vi "GradientVI.vi"(0 "x(m)":dbl[](array[numeric])=[-0.124, -0.174, 0.124, 0.174], 1 "erot(V/cm)":dbl=22.0, 5 "B(G)":dbl[](array[numeric])=[0.670549623135055, 0.512230952892665, 0.685842810963684, 0.53621930068775], 7 "uncertainty(G)":dbl[](array[numeric])=[0.010516573446927, 0.009705496604384, 0.010177056389311, 0.011331487675758], 9 "initial guess(A)":dbl[](array[numeric])=[0.5], 11 "error in (no error)":errorcluster, 12 "freq (Hz)":dbl=1589645.882716435) -> (4 "Fitted I(A)":dbl[](array[numeric])=[0.7805554383201968], 6 "dB(mG/cm)":dbl=66.15007442640399, 8 "Frequency(Hz)":dbl=35.75963864978995, 10 "XY Graph":cluster{"X":dbl[], "Y":dbl[]}[](graph)=[{"X"=[-0.2, -0.19798994974874373, -0.19597989949748745, -0.19396984924623117, -0.1919597989949749, -0.18994974874371862, -0.1879396984924623, -0.18592964824120603, -0.18391959798994975, -0.18190954773869347, -0.1798994974874372, -0.17788944723618091, -0.17587939698492464, -0.17386934673366836, -0.17185929648241208, -0.1698492462311558, -0.16783919597989952, -0.1658291457286432, -0.16381909547738693, -0.16180904522613065, -0.15979899497487438, -0.1577889447236181, -0.15577889447236182, -0.15376884422110554, -0.15175879396984926, -0.14974874371859298, -0.1477386934673367, -0.14572864321608042, -0.14371859296482412, -0.14170854271356784, -0.13969849246231156, -0.13768844221105528, -0.135678391959799, -0.13366834170854272, -0.13165829145728644, -0.12964824120603016, -0.12763819095477388, -0.1256281407035176, -0.12361809045226131, -0.12160804020100503, -0.11959798994974875, -0.11758793969849247, -0.11557788944723618, -0.1135678391959799, -0.11155778894472362, -0.10954773869346734, -0.10753768844221107, -0.10552763819095477, -0.1035175879396985, -0.10150753768844221, -0.09949748743718594, -0.09748743718592966, -0.09547738693467338, -0.09346733668341708, -0.0914572864321608, -0.08944723618090453, -0.08743718592964825, -0.08542713567839197, -0.08341708542713569, -0.0814070351758794, -0.07939698492462312, -0.07738693467336684, -0.07537688442211056, -0.07336683417085428, -0.07135678391959799, -0.06934673366834171, -0.06733668341708543, -0.06532663316582915, -0.06331658291457287, -0.061306532663316586, -0.05929648241206031, -0.05728643216080402, -0.05527638190954774, -0.05326633165829146, -0.05125628140703518, -0.0492462311557789, -0.04723618090452262, -0.04522613065326633, -0.043216080402010054, -0.04120603015075377, -0.03919597989949749, -0.03718592964824121, -0.035175879396984924, -0.033165829145728645, -0.031155778894472363, -0.02914572864321608, -0.0271356783919598, -0.02512562814070352, -0.023115577889447236, -0.021105527638190957, -0.019095477386934675, -0.017085427135678392, -0.015075376884422112, -0.01306532663316583, -0.011055276381909548, -0.009045226130653268, -0.007035175879396985, -0.005025125628140704, -0.0030150753768844224, -0.0010050251256281408, 0.0010050251256281408, 0.0030150753768844224, 0.005025125628140704, 0.007035175879396985, 0.009045226130653268, 0.011055276381909548, 0.01306532663316583, 0.015075376884422112, 0.017085427135678392, 0.019095477386934675, 0.021105527638190957, 0.023115577889447236, 0.02512562814070352, 0.0271356783919598, 0.02914572864321608, 0.031155778894472363, 0.033165829145728645, 0.035175879396984924, 0.03718592964824121, 0.03919597989949749, 0.04120603015075377, 0.043216080402010054, 0.04522613065326633, 0.04723618090452262, 0.0492462311557789, 0.05125628140703518, 0.05326633165829146, 0.05527638190954774, 0.05728643216080402, 0.05929648241206031, 0.061306532663316586, 0.06331658291457287, 0.06532663316582915, 0.06733668341708543, 0.06934673366834171, 0.07135678391959799, 0.07336683417085428, 0.07537688442211056, 0.07738693467336684, 0.07939698492462312, 0.0814070351758794, 0.08341708542713569, 0.08542713567839197, 0.08743718592964825, 0.08944723618090453, 0.0914572864321608, 0.09346733668341708, 0.09547738693467338, 0.09748743718592966, 0.09949748743718594, 0.10150753768844221, 0.1035175879396985, 0.10552763819095477, 0.10753768844221107, 0.10954773869346734, 0.11155778894472362, 0.1135678391959799, 0.11557788944723618, 0.11758793969849247, 0.11959798994974875, 0.12160804020100503, 0.12361809045226131, 0.1256281407035176, 0.12763819095477388, 0.12964824120603016, 0.13165829145728644, 0.13366834170854272, 0.135678391959799, 0.13768844221105528, 0.13969849246231156, 0.14170854271356784, 0.14371859296482412, 0.14572864321608042, 0.1477386934673367, 0.14974874371859298, 0.15175879396984926, 0.15376884422110554, 0.15577889447236182, 0.1577889447236181, 0.15979899497487438, 0.16180904522613065, 0.16381909547738693, 0.1658291457286432, 0.16783919597989952, 0.1698492462311558, 0.17185929648241208, 0.17386934673366836, 0.17587939698492464, 0.17788944723618091, 0.1798994974874372, 0.18190954773869347, 0.18391959798994975, 0.18592964824120603, 0.1879396984924623, 0.18994974874371862, 0.1919597989949749, 0.19396984924623117, 0.19597989949748745, 0.19798994974874373, 0.2], "Y"=[0.4343731207716029, 0.4433656420187343, 0.4523999073237652, 0.4614632556723153, 0.4705421469697098, 0.47962216308459116, 0.48868801544118295, 0.49772355973172244, 0.5067118182846725, 0.515635010574119, 0.5244745922903558, 0.5332113033105923, 0.5418252248117672, 0.5502958456549943, 0.558602138043926, 0.5667226423186786, 0.5746355605948373, 0.5823188587959173, 0.5897503764606421, 0.5969079435370565, 0.6037695032079631, 0.6103132396308245, 0.61651770932489, 0.6223619748035435, 0.627825738935488, 0.6328894784287399, 0.6375345747704844, 0.6417434409268228, 0.6454996421119438, 0.648788008977546, 0.6515947416510275, 0.653907503164066, 0.6557155009600026, 0.6570095553456443, 0.6577821539567437, 0.65802749153128, 0.6577414945251566, 0.6569218303545473, 0.6555679013014879, 0.6536808233676547, 0.6512633905993845, 0.6483200256288755, 0.6448567173770191, 0.6408809470380492, 0.6364016036117994, 0.6314288903634748, 0.6259742236722772, 0.6200501257787339, 0.6136701129570843, 0.6068485806252242, 0.5996006868630789, 0.5919422357439666, 0.5838895617961289, 0.5754594168070625, 0.5666688600656038, 0.557535153009968, 0.5480756591180211, 0.5383077497426845, 0.5282487164638761, 0.5179156904018862, 0.5073255688180945, 0.4964949492198238, 0.48544007108869297, 0.474176765267704, 0.462720410972733, 0.45108590034032897, 0.439287610386756, 0.42733938223441237, 0.41525450746244597, 0.4030457214608077, 0.3907252037138467, 0.3783045850151782, 0.3657949617259116, 0.3532069173422856, 0.3405505518490638, 0.327835519620349, 0.31507107701690007, 0.3022661413586166, 0.28942936368165795, 0.2765692187103993, 0.2636941169192627, 0.25081254563422967, 0.2379332491492377, 0.22506546231523405, 0.21221921881361852, 0.19940576568118554, 0.1866381318219849, 0.17393192396203172, 0.16130646520063135, 0.14878646017219702, 0.13640448646158432, 0.12420480847971814, 0.11224934499071332, 0.10062718140932637, 0.08946988768293114, 0.07897595414571017, 0.06944764758546348, 0.06133726668859257, 0.05527294501450065, 0.051976078966787596, 0.051976077274574824, 0.05527294024070014, 0.061337259519021615, 0.06944763872056539, 0.07897594412364949, 0.08946987687137098, 0.1006271700501765, 0.11224933324318014, 0.12420479645040532, 0.13640447422365204, 0.14878644777724576, 0.16130645268611501, 0.17393191135594288, 0.18663811914589734, 0.1994057529522514, 0.21221920604592923, 0.22506544952075688, 0.2379332363384778, 0.25081253281671645, 0.26369410410389543, 0.27656920590571804, 0.2894293508960435, 0.3022661286004478, 0.31507106429468024, 0.32783550694280555, 0.34055053922522777, 0.3532069047815553, 0.3657949492381077, 0.37830457261058625, 0.3907251914032473, 0.4030457092555054, 0.415254495374284, 0.4273393702757855, 0.43928759857061345, 0.45108588868017013, 0.4627203994826003, 0.4741767539621622, 0.48544005998280776, 0.4964949383291282, 0.5073255581585516, 0.5179156799898412, 0.5282487063160028, 0.5383077398759236, 0.5480756495495115, 0.5575351437569672, 0.5666688511454083, 0.5754594082369142, 0.5838895535931194, 0.5919422279249344, 0.5996006794445035, 0.6068485736231135, 0.6136701063868614, 0.6200501196551201, 0.6259742180091787, 0.6314288851738644, 0.6364015989076046, 0.6408809428300443, 0.6448567136747175, 0.6483200224404359, 0.6512633879315217, 0.6536808212255597, 0.6555678996887611, 0.6569218292731409, 0.6577414939753324, 0.6580274915115836, 0.6577821544639861, 0.6570095563749091, 0.6557155025046587, 0.653907505215802, 0.6515947441998958, 0.6487880120120281, 0.645499645619021, 0.6417434448920682, 0.6375345791781551, 0.632889483261892, 0.6278257441760874, 0.6223619804325953, 0.616517715322559, 0.6103132459765754, 0.6037695098806889, 0.5969079505152144, 0.5897503837223826, 0.5823188663192184, 0.5746355683576233, 0.5667226502989444, 0.5586021462198473, 0.5502958540050344, 0.5418252333147743, 0.5332113119458863, 0.5244746010378123, 0.5156350194142353, 0.5067118271986327, 0.497723568701447, 0.48868802444937526, 0.4796221721147673, 0.47054215600622995, 0.4614632647003972, 0.45239991632950055, 0.4433656509890871, 0.43437312969441233]}, {"X"=[-0.124, -0.174, 0.124, 0.174], "Y"=[0.670549623135055, 0.512230952892665, 0.685842810963684, 0.53621930068775]}], 15 "error out":errorcluster)   [LabVIEW 2012]
uses:
  <vilib>/Analysis/1siggen.llb/Ramp Pattern by Samples.vi
  <vilib>/Analysis/NI_AALBase.lvlib
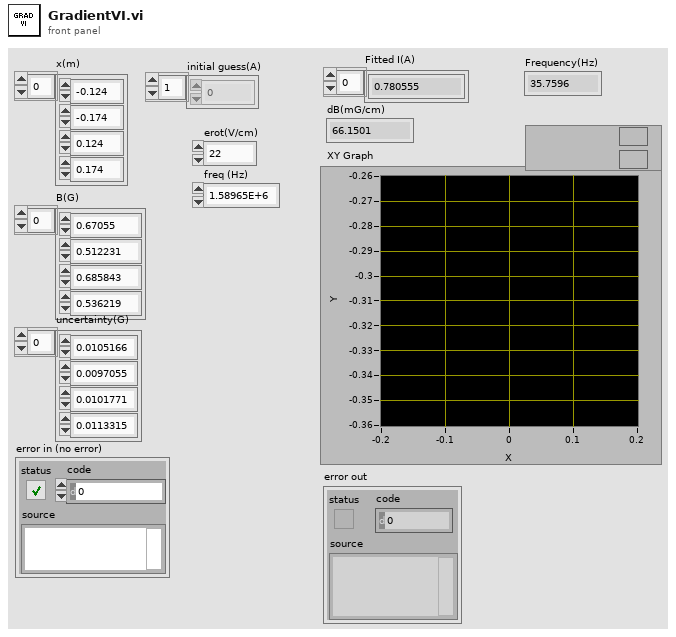
[diagram p1: front panel]
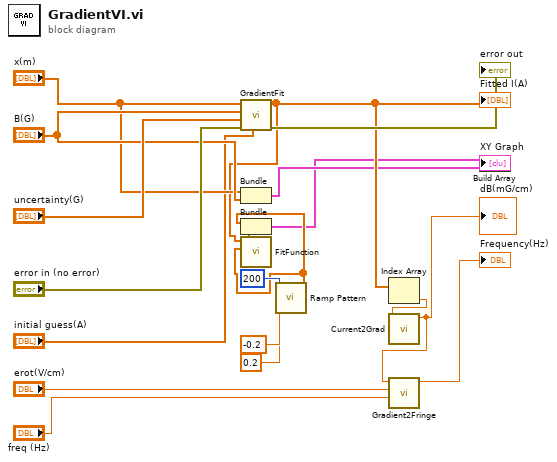
[diagram p0: block diagram]
diagram:
  n1 = call "GradientFit.vi"("initial parameters(A)"="initial guess(A)", "error in (no error)"="error in (no error)", "uncertainty"="uncertainty(G)", "B(G)"="B(G)", "x(m)"="x(m)") -> ("error out"=→"error out":errorcluster, "Fitted I(A)"=w8:dbl[])  [unwired: 5 in]
  "Fitted I(A)" <- w8
  n2 = Bundle("x(m)"="x(m)", "B(G)"="B(G)") -> (w2:cluster{"x(m)":dbl[], "B(G)":dbl[]})  [unwired: 1 in]
  n3 = call-poly <vilib>:"Ramp Pattern.vi"("start"=-0.2, "end"=0.2, "samples"=200) -> ("Ramp Pattern"=w10:dbl[])  [unwired: 7 in, 1 out]
  n4 = call "FitFunction.vi"("X"=w10, "a"=w8) -> ("f(X,a)(G)"=w16:dbl[])  [unwired: 2 in, 2 out]
  n5 = Bundle("Ramp Pattern"=w10, "f(X,a)(G)"=w16) -> (w1:cluster{"Ramp Pattern":dbl[], "f(X,a)(G)":dbl[]})  [unwired: 1 in]
  n6 = Index Array(array=w8) -> (element=w7:dbl)  [unwired: 1 in]
  n7 = call "Current2Grad.vi"("I(A)"=w7) -> ("dB(mG/cm)"=w6:dbl)  [unwired: 10 in]
  "dB(mG/cm)" <- w6
  n8 = call "Gradient2Fringe.vi"("freq (Hz)"="freq (Hz)", "erot(V/cm)"="erot(V/cm)", "dB(mG/cm)"=w6) -> ("Frequency(Hz)"=→"Frequency(Hz)":dbl)  [unwired: 8 in]
  n9 = Build Array(w1, w2) -> (→"XY Graph":cluster{"x(m)":dbl[], "B(G)":dbl[]}[])
